vi "RIS.vi"(2 "Run uninterrupted?":bool, 3 "Device Category IN:":string(combo)="Short Strip" caption="Device Category:", 4 "Structure:":string, 5 "DB Serial No.:":string, 6 "Sensor Serial No.:":string) -> (0 "Done!":bool)   [LabVIEW 2019]
doc: "Performs Ris measurements according to ATLAS ITk Quality Control Specifications."
uses:
  <vilib>/Analysis/6fits.llb/Curve Fitting Criteria.ctl
  general_VIs/globals/QC_MeasurementSetup.vi
  general_VIs/globals/QC_RunInformation.vi
  InstrControl/InstrumentSetup.vi
  InstrControl/Switching/Switching.lvclass
  InstrControl/SupplyControl/SupplyControl.lvclass
  InstrControl/MultimeterControl/MultimeterControl.lvclass
  InstrControl/ArduinoControl/ArduinoControl.lvclass
  <vilib>/Analysis/NI_AALBase.lvlib
  InstrControl/InstrControl.lvclass
  <vilib>/Analysis/NI_AALPro.lvlib
panel:
  out "Ris":dbl[](array[numeric]) caption="Ris [MOhm]"
  out "Volts":dbl[](array[numeric]) caption="Volts [V]"
  out "Current":dbl[](array[numeric]) caption="Current [nA]"
  in  "No. of readouts":i32=5
  out "Risgraph":cluster{dbl[], dbl[]}(graph)
  out "Vigraph":cluster{i32[], dbl[]}[](graph)
  out "Imgraph":cluster{i32[], dbl[]}[](graph)
  in  "Initial volts [V]":dbl format="%.1f"
  in  "Final volts [V]":dbl=-700.0 format="%.1f"
  in  "step [V]":dbl=10.0 format="%.1f"
  in  "step interval [s]":u32=10
  out "Temp.":dbl[](array[numeric]) caption="Temp. [°C]" format="%#.2f"
  out "RH":dbl[](array[numeric]) caption="RH [%]" format="%#.2f"
  out "positive ramp?":bool
  out "Tab Control":enum32{"Ris Setup", "Ris Scan"}(tab)
  in  "Switching":string(combo)="Pickering Matrix"
  in  "Voltmeter":string(combo)="HP34401A"
  in  "Ris SMU":string(combo)="Keithley 2657A"
  in  "Current Limit [µA]":dbl=20.0 min=0.0001 format="%.3f"
  in  "Set\ncurrent\nlimit?":bool
  in  "Temperature":enum16{"Read Arduino", "Enter manually"}(ring)
  in  "Ris Supply":string(combo)="Keithley 2410"
  in  "User:":string(combo)="Graham"
  in  "Manufacturer:":string(combo)="Hamamatsu"
  in  "Quit":bool
  in  "Continue":bool
  in  "abort":bool
  out "Device Category:":string
  out "DB Serial Number:":string
  out "Current Volts:":dbl format="%.2f"
  in  "quit (no save)":bool
  in  "Quit & Save":bool
  out "Bias On/Off:":bool
  out "STATUS 1":string
  out "Initiated:":string
  out "Sensor No.:":string
  out "No of steps":u32
  out "Current reading No.":u32
  out "Last reading at:":string
  out "Ris SMU Current [nA]":dbl[][][](array[numeric])
  out "Ris induced Voltage [V]":dbl[][][](array[numeric])
  # "University of\nCambridge"
  # "Strip Sensor QC: inter-strip Resistance"
  # "Ris Scan parameters:"
  # "Last 5 readings:"
  # "n-4"
  # "n-3"
  # "n-2"
  # "n-1"
  # "n"
  # "DUT & Test Description"
  # "Hardware"
  # "DUT & Test Description:"
  # "Current status:"
  # "Rdg No:"
  # "out of"
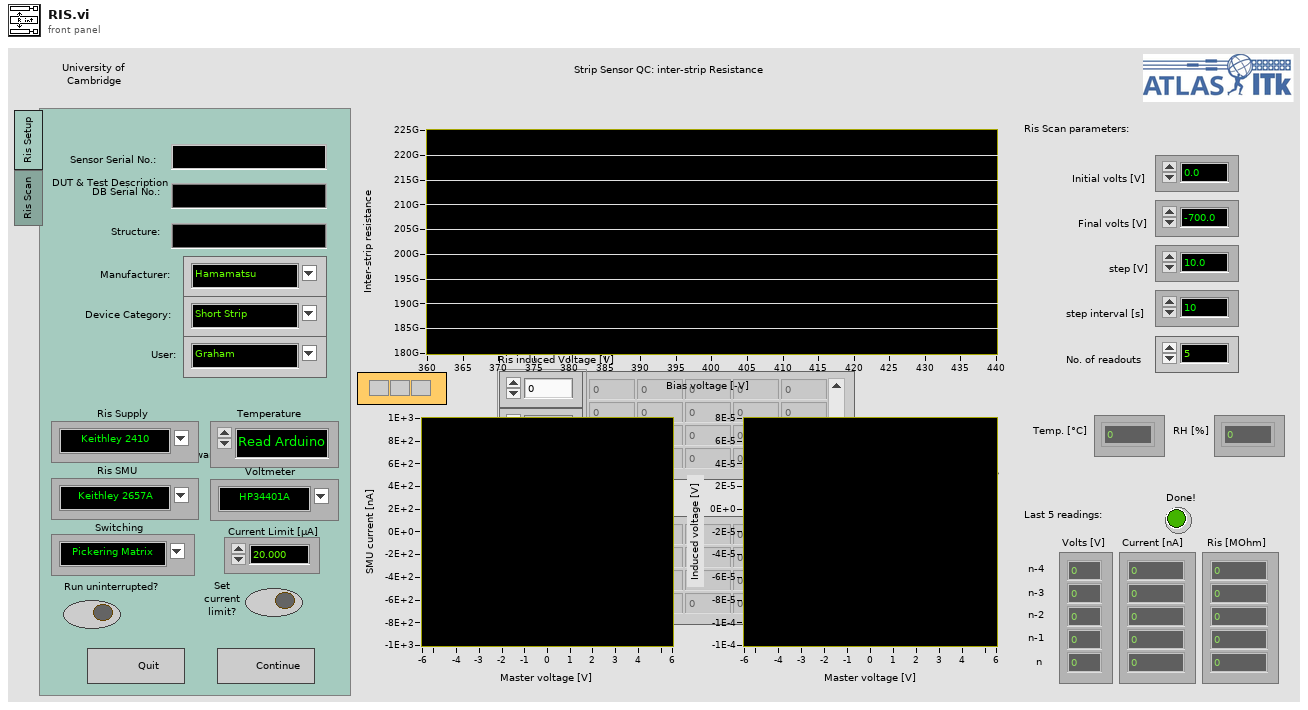
[diagram p1: front panel]
types:
  T1 = enum16{"Supply", "LCR", "Multimeter", "Switching"}
  T2 = enum16{"Reset", "Read Array", "Read Element", "Write Element", "Write Array", "Add Element", "Add Array"}
  T3 = enum16{"Reset", "Ground", "Striptest Bias", "Striptest SMU", "Striptest LCR", "IV", "CV", "Interstrip Cap", "Interstrip Res"}
  T4 = enum16{"Reset", "Ground", "Striptest Bias", "Striptest SMU", "Striptest LCR", "IV", "CV", "Interstrip Cap", "Interstrip Res", "PTP", "Implant Resistance", "Metal Resistance", "Coupling Capacitance"}
  T5 = enum32{"IV", "CV", "Stability", "Striptest", "Cis", "Ris", "PTP"}
  T6 = cluster{"Sensor Serial No.:":string, "Wafer Serial No.:":string, "Batch:":string, "Manufacturer:":string, "Device Category:":string, "Database Serial No.:":string, "Date Initiated:":string, "Time Initiated:":string, "Test":string, "Instruments used:":string, "Probeplan used:":string, "End of Run comment:":string, "User:":string}
  T7 = cluster{"Institute":string, "Manufacturers":string[], "Devices":string[], "Serialnumbers Lookup DB":string, "Data directory":string, "Backup & screenshot directory":string, "List of known users":string[], "Measurement switch not used":bool, "Measurement Switch":string, "DUT Switch":string}
  T8 = cluster{"Bias Supply":refnum<class "SupplyControl.lvclass">, "SMU":refnum<class "SupplyControl.lvclass">, "Multimeter":refnum<class "MultimeterControl.lvclass">, "Initial Voltage [V]":dbl, "Final Voltage [V]":dbl, "Step Size [V]":dbl, "Step Interval [s]":i32, "Number Of Steps":u32, "Ramp down steps [V]":dbl, "Ramp down Interval [s]":i32, "Set Current Limit?":bool, "Current Limit [µA]":dbl, "Temperature Readout":enum16{"Read Arduino", "Enter manually"}, "Arduino":refnum<class "ArduinoControl.lvclass">, "Supply Name":string, "SMU Name":string, "Voltmeter Name":string, "R_is Limit [MOhm]":dbl, "Switching":refnum<class "Switching.lvclass">, "Matrix used?":bool, "Matrix X Channels":cluster{"Bias Supply / SMU LO":i32, "Bias Supply / SMU HI":i32, "CV Box LO":i32, "CV Box HI":i32, "CV Box LO IN":i32, "CV Box HI IN":i32, "Volt meter LO":i32, "Volt meter HI":i32, "Mux1 C1":i32, "Mux1 C2":i32, "Mux2 C1":i32, "Mux2 C2":i32}, "Structure Name":string}
  T9 = cluster{"Current Limit":sgl, "KE2410":refnum<class "KE2410.lvclass">}
  T10 = cluster{"VISA address":refnum<visa-resource-name>, "T sensor":enum16{"SHT", "DS"}, "Arduino":refnum<class "ArduinoControl.lvclass">}
  T11 = typedef "NI_AALPro.lvlib/Curve Fitting Criteria.ctl" = u16
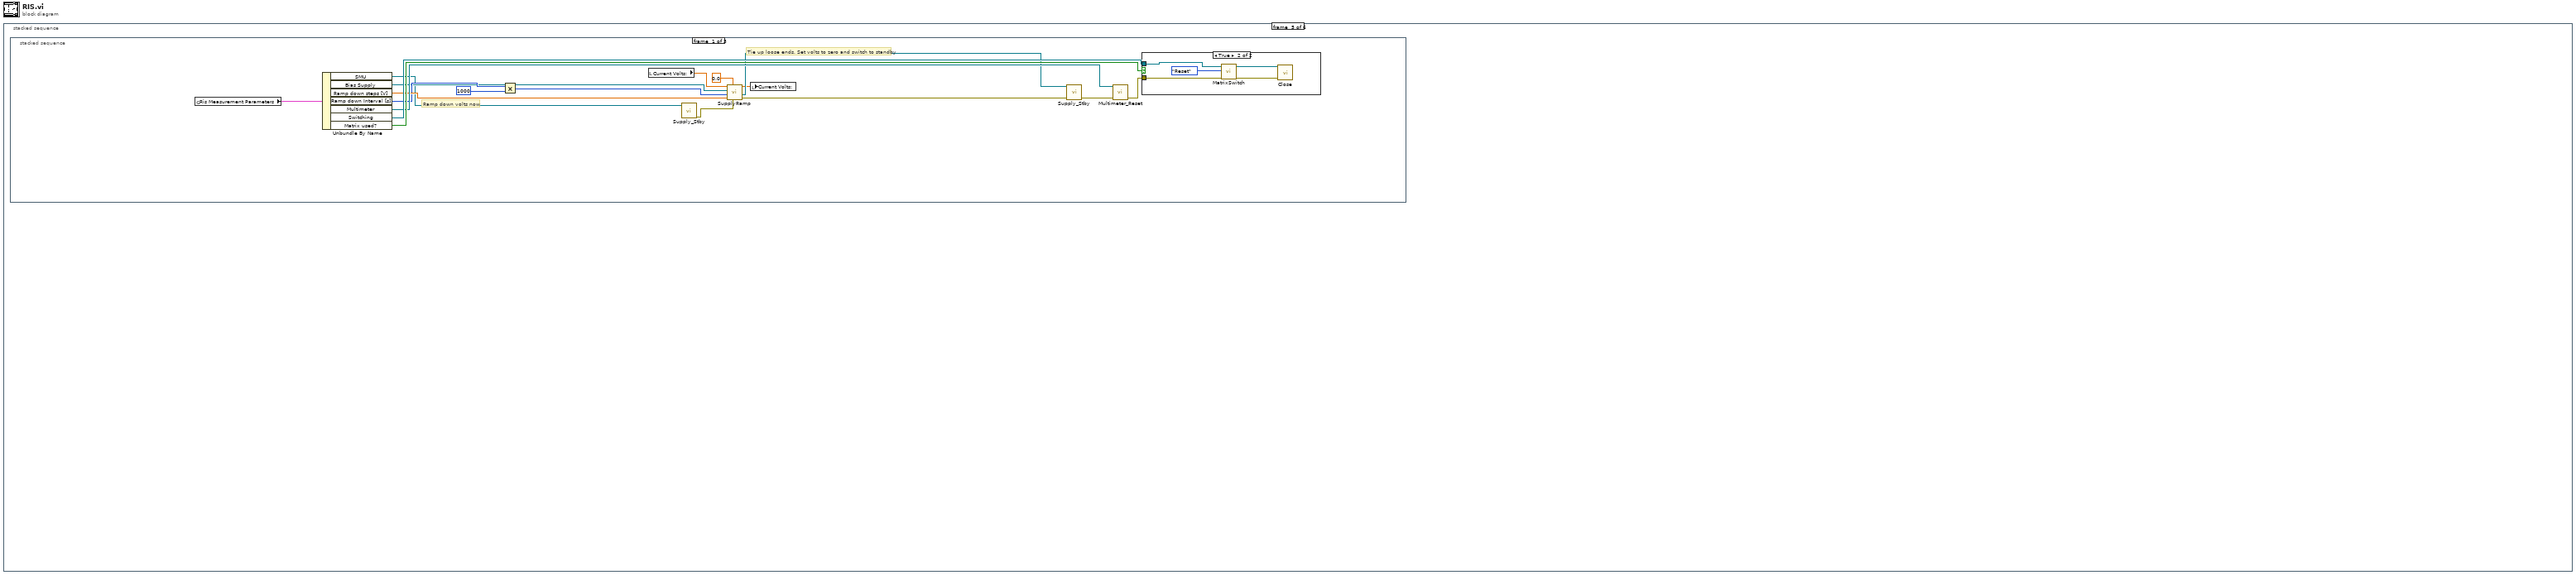
[diagram p0: block diagram]
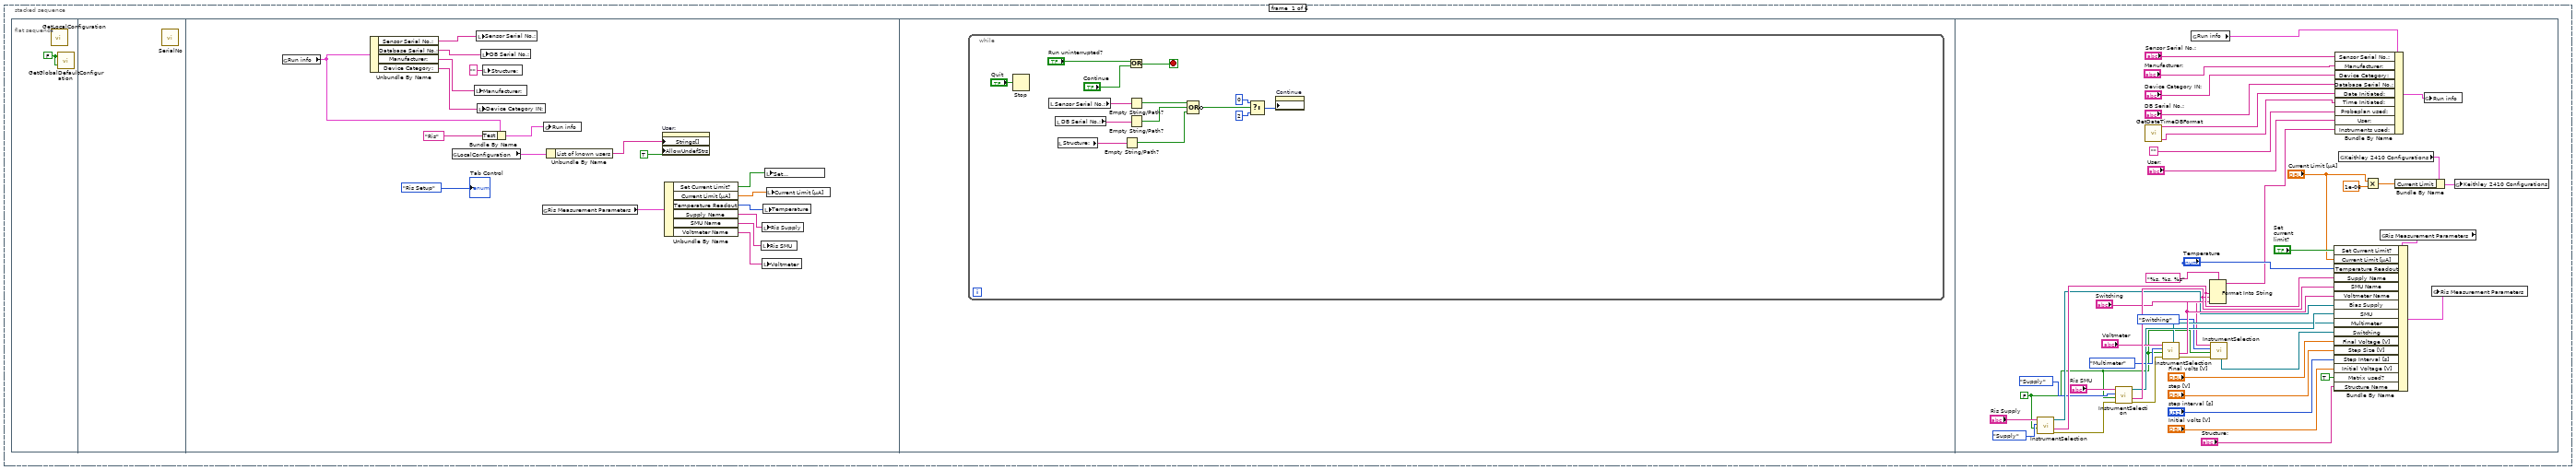
[diagram p2: hidden frame]
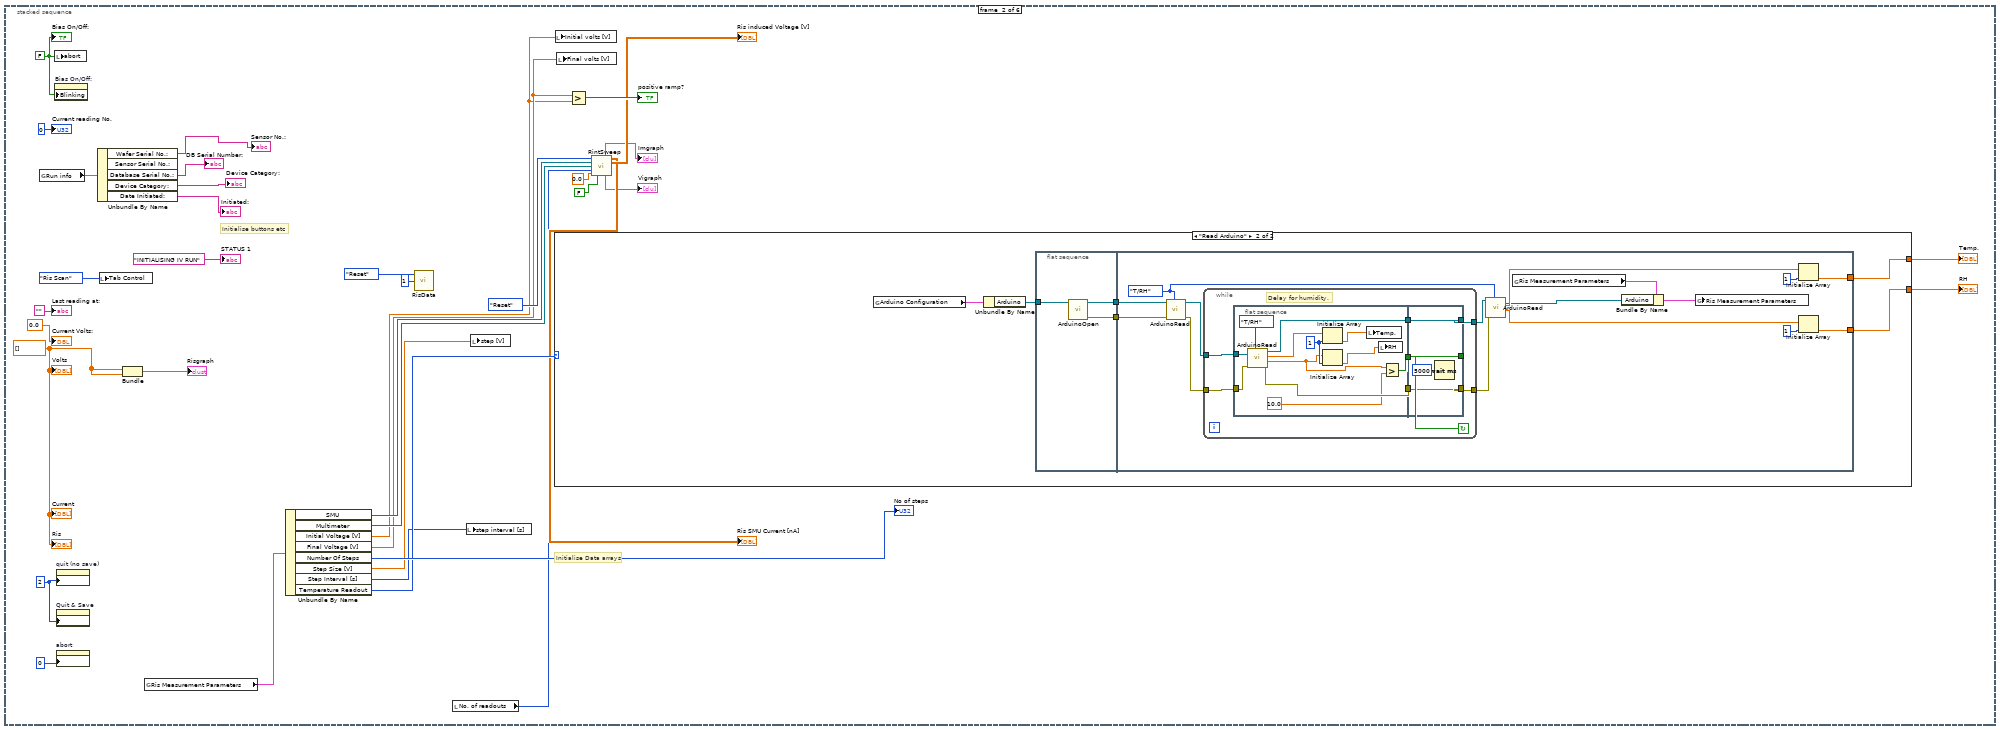
[diagram p3: hidden frame]
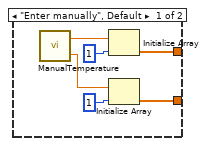
[diagram p4: hidden frame]
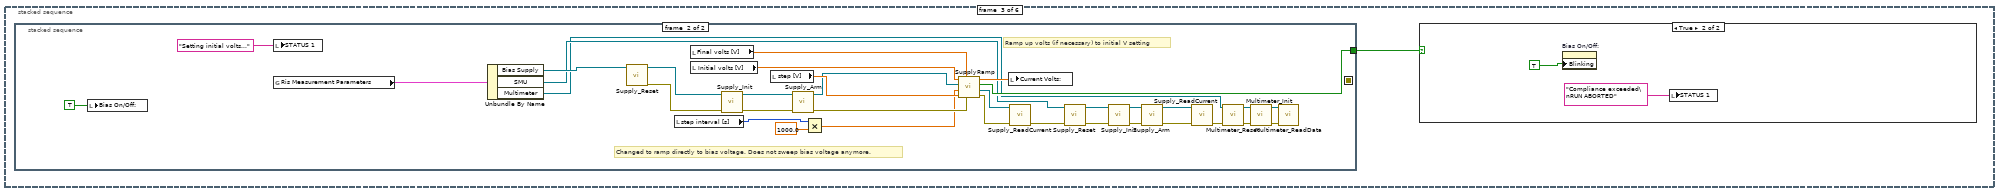
[diagram p5: hidden frame]
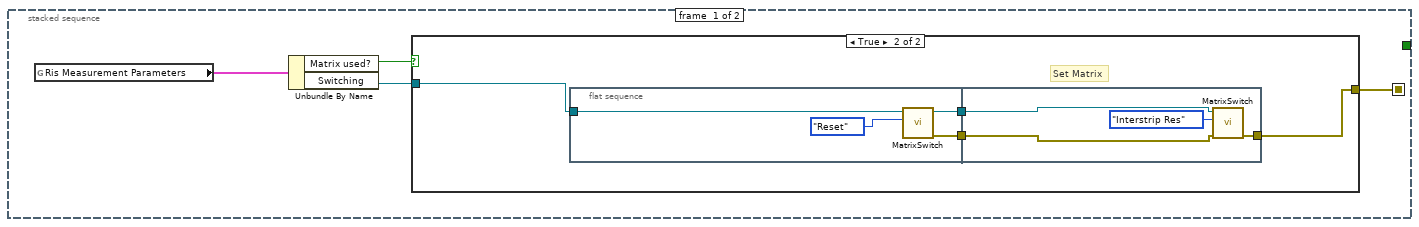
[diagram p6: hidden frame]
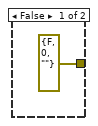
[diagram p7: hidden frame]
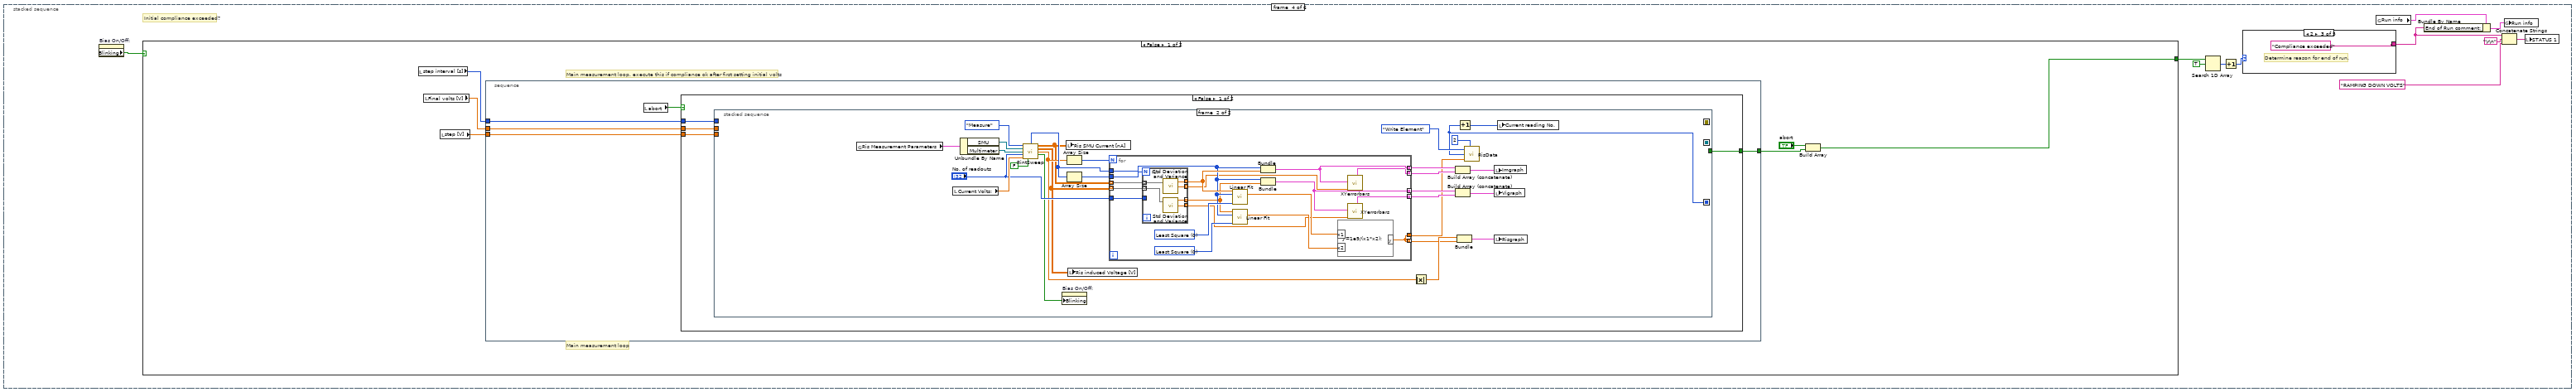
[diagram p9: hidden frame]
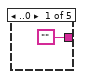
[diagram p10: hidden frame]
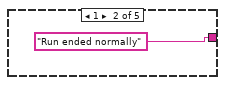
[diagram p11: hidden frame]
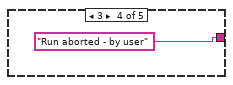
[diagram p12: hidden frame]
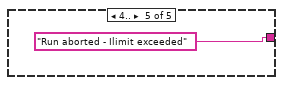
[diagram p13: hidden frame]
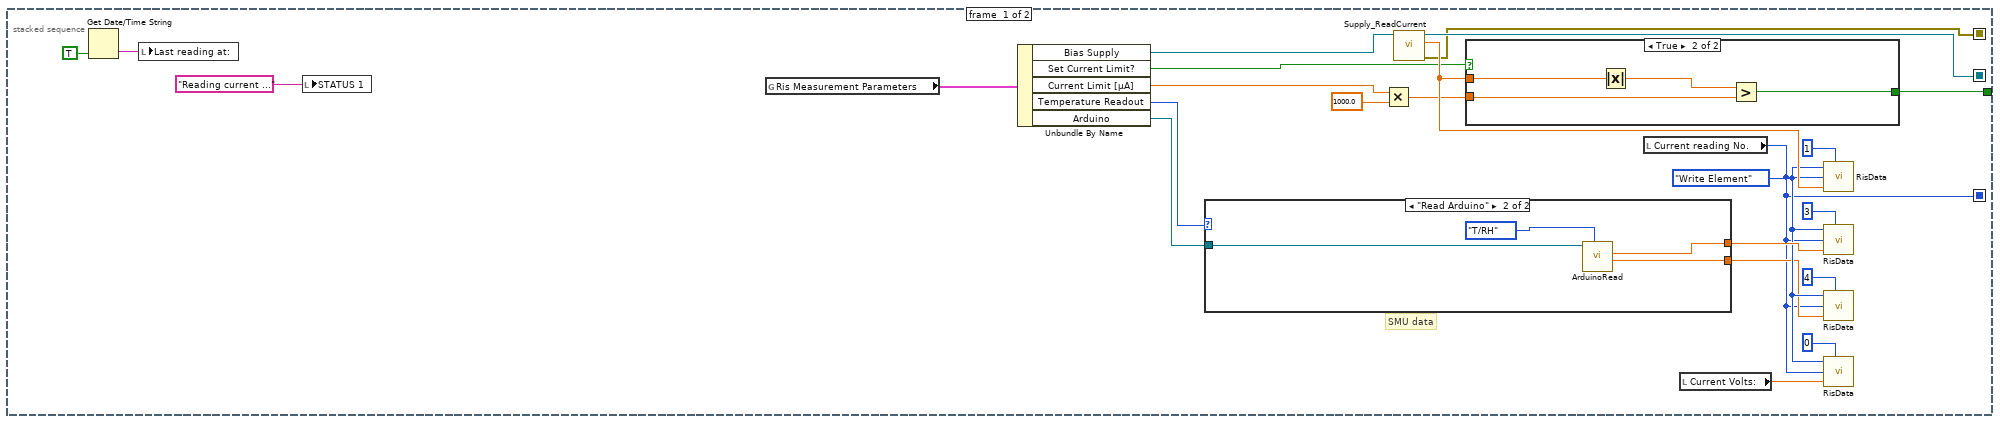
[diagram p14: hidden frame]
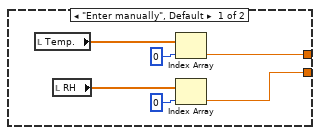
[diagram p15: hidden frame]
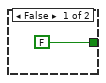
[diagram p16: hidden frame]
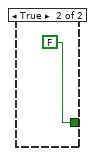
[diagram p17: hidden frame]
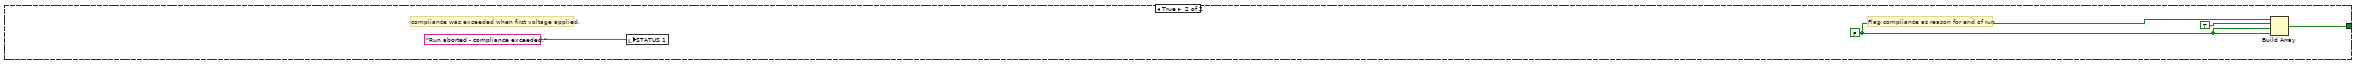
[diagram p18: hidden frame]
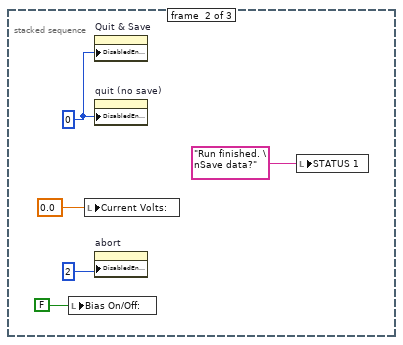
[diagram p20: hidden frame]
diagram:
  n1 = stacked-sequence {
    frame #0 {
      n2 = flat-sequence {
        frame #0 {
          w1 = FALSE
          n3 = call "GetLocalConfiguration.vi"() -> ()  [unwired: 3 in, 1 out]
          n4 = call "GetGlobalDefaultConfiguration.vi"("DO NOT override instruments"=w1, "Read defaults?"=w1) -> ()  [unwired: 1 in, 1 out]
        }
        frame #1 {
          n5 = call "SerialNo.vi"() -> ()  [unwired: 5 in, 1 out]
        }
        frame #2 {
          n6 = global read "QC_RunInformation.vi" "Run info"() -> (w7:T6)
          n7 = Unbundle By Name(w7) -> ("Sensor Serial No.:"=w4:string, "Database Serial No.:"=w5:string, "Manufacturer:"=w3:string, "Device Category:"=w6:string)
          n8 = global read "QC_RunInformation.vi" "LocalConfiguration"() -> (w15:T7)
          n9 = local write "Manufacturer:"(w3) -> ()
          n10 = local write "Sensor Serial No.:"(w4) -> ()
          n11 = local write "Device Category IN:"(w6) -> ()
          n12 = local write "DB Serial No.:"(w5) -> ()
          n13 = local write "Structure:"("" ("Structure:")) -> ()
          n14 = Bundle By Name(cluster=w7, "Test"="Ris") -> (w12:T6)
          n15 = global read "QC_MeasurementSetup.vi" "Ris Measurement Parameters"() -> (w18:T8)
          n16 = global write "QC_RunInformation.vi" "Run info"(w12) -> ()
          n17 = Unbundle By Name(w15) -> ("List of known users"=w14:string[])
          n18 = property on="User:" class="CmbBox"("Strings[]"=w14, "AllowUndefStrs"=TRUE) -> ()  [unwired: 2 in, 2 out]
          n19 = Unbundle By Name(w18) -> ("Set Current Limit?"=w17:bool, "Current Limit [µA]"=w16:dbl, "Temperature Readout"=w20:enum16{"Read Arduino", "Enter manually"}, "Supply Name"=w19:string, "SMU Name"=w9:string, "Voltmeter Name"=w8:string)
          n20 = local write "Ris SMU"(w9) -> ()
          n21 = local write "Ris Supply"(w19) -> ()
          n22 = local write "Voltmeter"(w8) -> ()
          n23 = local write "Temperature"(w20) -> ()
          n24 = local write "Set\ncurrent\nlimit?"(w17) -> ()
          n25 = local write "Current Limit [µA]"(w16) -> ()
          "Tab Control" <- enum32{"Ris Setup", "Ris Scan"}."Ris Setup" ("Tab Control")
        }
        frame #3 {
          n26 = while {
            stop <- w23 stop-if-true
            n27 = Stop(stop? (T)="Quit") -> ()
            n28 = local read "Sensor Serial No.:"() -> (w33:string)
            n29 = local read "DB Serial No.:"() -> (w32:string)
            n30 = local read "Structure:"() -> (w22:string)
            n31 = Empty String/Path?(string/path=w22) -> (empty?=w21:bool)
            n32 = Or(x="Run uninterrupted?", y="Continue") -> (x .or. y?=w23:bool)
            n33 = Empty String/Path?(string/path=w33) -> (empty?=w30:bool)
            n34 = Empty String/Path?(string/path=w32) -> (empty?=w31:bool)
            n35 = Compound Arithmetic op=OR(w30, w31, w21) -> (invert w29:bool)
            n36 = Select(t=0, s=w29, f=2) -> (s? t:f=w26:i32)
            n37 = property on="Continue" class="Bool"("DisabledEnum"=w26) -> ()  [unwired: 2 in, 2 out]
          }
        }
        frame #4 {
          w52 = FALSE
          n38 = call "InstrumentSelection.vi"("Verify GPIB address"=w52, "Instrument type"=T1."Supply", "Instrument name IN"="Ris Supply") -> ("error out"=w59:errorcluster, "Instrument name OUT"=w67:string, "Supply"=w62:refnum<class "SupplyControl.lvclass">)  [unwired: 3 in, 3 out]
          n39 = call "InstrumentSelection.vi"("error in (no error)"=w59, "Verify GPIB address"=w52, "Instrument type"=T1."Supply", "Instrument name IN"="Ris SMU") -> ("error out"=w58:errorcluster, "Instrument name OUT"=w65:string, "Supply"=w61:refnum<class "SupplyControl.lvclass">)  [unwired: 2 in, 3 out]
          n40 = call "GetDateTimeDBFormat.vi"() -> ("Time in 24h format, e.g. 13:40:54"=w36:string, "Abbreviated Date, e.g. 13 Nov 2020"=w38:string)  [unwired: 10 in]
          n41 = call "InstrumentSelection.vi"("error in (no error)"=w58, "Verify GPIB address"=w52, "Instrument type"=T1."Multimeter", "Instrument name IN"="Voltmeter") -> ("error out"=w57:errorcluster, "Instrument name OUT"=w63:string, "Multimeter"=w60:refnum<class "MultimeterControl.lvclass">)  [unwired: 2 in, 3 out]
          n42 = global read "QC_RunInformation.vi" "Run info"() -> (w78:T6)
          n43 = Format Into String(format string="%s, %s, %s", w67, w65, w63) -> (resulting string=w35:string)  [unwired: 2 in, 1 out]
          n44 = call "InstrumentSelection.vi"("error in (no error)"=w57, "Verify GPIB address"=w52, "Instrument type"=T1."Switching", "Instrument name IN"="Switching") -> ("Switching"=w51:refnum<class "Switching.lvclass">)  [unwired: 2 in, 5 out]
          n45 = Bundle By Name(cluster=w78, "Sensor Serial No.:"="Sensor Serial No.:", "Manufacturer:"="Manufacturer:", "Device Category:"="Device Category IN:", "Database Serial No.:"="DB Serial No.:", "Date Initiated:"=w38, "Time Initiated:"=w36, "Probeplan used:"="", "User:"="User:", "Instruments used:"=w35) -> (w77:T6)
          n46 = global read "InstrumentSetup.vi" "Keithley 2410 Configurations"() -> (w43:T9)
          n47 = Multiply(x="Current Limit [µA]", y=1e-06) -> (x*y=w40:dbl)
          n48 = global read "QC_MeasurementSetup.vi" "Ris Measurement Parameters"() -> (w79:T8)
          n49 = Bundle By Name(cluster=w79, "Set Current Limit?"="Set\ncurrent\nlimit?", "Current Limit [µA]"="Current Limit [µA]", "Temperature Readout"="Temperature", "Supply Name"=w67, "SMU Name"=w65, "Voltmeter Name"=w63, "Bias Supply"=w62, "SMU"=w61, "Multimeter"=w60, "Switching"=w51, "Final Voltage [V]"="Final volts [V]", "Step Size [V]"="step [V]", "Step Interval [s]"="step interval [s]", "Initial Voltage [V]"="Initial volts [V]", "Matrix used?"=TRUE, "Structure Name"="Structure:") -> (w80:T8)
          n50 = Bundle By Name(cluster=w43, "Current Limit"=w40) -> (w44:T9)
          n51 = global write "QC_RunInformation.vi" "Run info"(w77) -> ()
          n52 = global write "QC_MeasurementSetup.vi" "Ris Measurement Parameters"(w80) -> ()
          n53 = global write "InstrumentSetup.vi" "Keithley 2410 Configurations"(w44) -> ()
        }
      }
    }
    frame #1 {
      w92 = dbl[] []
      w108 = 2
      w107 = FALSE ("Visible")
      # "Initialise buttons etc"
      # "Initialise Data arrays"
      n54 = global read "QC_RunInformation.vi" "Run info"() -> (w116:T6)
      n55 = local write "abort"(w107) -> ()
      n56 = property on="Bias On/Off:" class="Bool (strict)"("Blinking"=w107) -> ()  [unwired: 2 in, 2 out]
      n57 = property on="quit (no save)" class="Bool"("DisabledEnum"=w108) -> ()  [unwired: 2 in, 2 out]
      n58 = property on="Quit & Save" class="Bool"("DisabledEnum"=w108) -> ()  [unwired: 2 in, 2 out]
      n59 = property on="abort" class="Bool (strict)"("DisabledEnum"=0) -> ()  [unwired: 2 in, 2 out]
      n60 = Unbundle By Name(w116) -> ("Wafer Serial No.:"=→"Sensor No.:":string, "Database Serial No.:"=→"DB Serial Number:":string, "Device Category:"=→"Device Category:":string, "Date Initiated:"=→"Initiated:":string)  [unwired: 1 out]
      n61 = local write "Tab Control"(enum32{"Ris Setup", "Ris Scan"}."Ris Scan" ("Tab Control")) -> ()
      n62 = Bundle(w92, w92) -> (→"Risgraph":cluster{dbl[], dbl[]})  [unwired: 1 in]
      n63 = global read "QC_MeasurementSetup.vi" "Ris Measurement Parameters"() -> (w103:T8)
      n64 = Unbundle By Name(w103) -> ("SMU"=w88:refnum<class "SupplyControl.lvclass">, "Multimeter"=w87:refnum<class "MultimeterControl.lvclass">, "Initial Voltage [V]"=w83:dbl, "Final Voltage [V]"=w84:dbl, "Number Of Steps"=→"No of steps":u32, "Step Size [V]"=w85:dbl, "Step Interval [s]"=w86:i32, "Temperature Readout"=w109:enum16{"Read Arduino", "Enter manually"})
      n65 = call "RisData.vi"("Action"=T2."Reset", "Array Size / Index"=u32 1) -> ()  [unwired: 3 in, 2 out]
      n66 = local read "No. of readouts"() -> (w90:i32)
      n67 = local write "step interval [s]"(w86) -> ()
      n68 = local write "step [V]"(w85) -> ()
      n69 = case shown="\"Read Arduino\"" w109 {
        tunnel: [w122 w129] -> w111
        tunnel: [w119 w128] -> w104
        frame "Enter manually", Default {
          n70 = call "ManualTemperature.vi"() -> ("Humidity [%] out"=w118:dbl, "Temperature [°C] out"=w123:dbl)
          n71 = Initialize Array(w123, 1) -> (w122:dbl[])
          n72 = Initialize Array(w118, 1) -> (w119:dbl[])
        }
        frame "Read Arduino" {
          n73 = global read "InstrumentSetup.vi" "Arduino Configuration"() -> (w125:T10)
          n74 = Unbundle By Name(w125) -> ("Arduino"=w124:refnum<class "ArduinoControl.lvclass">)
          n75 = flat-sequence {
            tunnel: [w130] -> w127
            tunnel: [w132] -> w126
            tunnel: w124 -> [w131]
            tunnel: [w148] -> w129
            tunnel: [w145] -> w128
            tunnel: w127 -> [w139]
            tunnel: w126 -> [w138]
            frame #0 {
              n76 = call "ArduinoOpen.vi"("ArduinoControl in"=w131) -> ("error out"=w132:errorcluster, "ArduinoControl out"=w130:refnum<class "ArduinoControl.lvclass">)  [unwired: 9 in]
            }
            frame #1 {
              w137 = enum16{"T/RH", "Interlock", "Edgesense"}."T/RH" ("Arduino function")
              n77 = call "ArduinoRead.vi"("Arduino function"=w137, "error in (no error)"=w138, "ArduinoControl in"=w139) -> ("error out"=w135:errorcluster, "ArduinoControl out"=w136:refnum<class "ArduinoControl.lvclass">)  [unwired: 3 in, 4 out]
              n78 = while {
                tunnel: w136 -> [w156]
                tunnel: w135 -> [w155]
                tunnel: [w153] -> w134
                tunnel: [w152] -> w133
                stop <- w154 continue-if-true
                # "Delay for humidity."
                n79 = flat-sequence {
                  tunnel: w156 -> [w168]
                  tunnel: w155 -> [w166]
                  tunnel: [w165] -> w151
                  tunnel: [w164] -> w150
                  tunnel: [w163] -> w149
                  tunnel: [w170] -> w152
                  tunnel: [w171] -> w153
                  tunnel: [w172] -> w154
                  tunnel: w151 -> [w172]
                  tunnel: w150 -> [w171]
                  tunnel: w149 -> [w170]
                  frame #0 {
                    w161 = 1
                    n80 = call "ArduinoRead.vi"("Arduino function"=enum16{"T/RH", "Interlock", "Edgesense"}."T/RH", "error in (no error)"=w166, "ArduinoControl in"=w168) -> ("error out"=w163:errorcluster, "rel. Humidity [%]"=w158:dbl, "Temperature [°C]"=w159:dbl, "ArduinoControl out"=w164:refnum<class "ArduinoControl.lvclass">)  [unwired: 3 in, 2 out]
                    n81 = Initialize Array(w159, w161) -> (w160:dbl[])
                    n82 = Initialize Array(w158, w161) -> (w157:dbl[])
                    n83 = local write "Temp."(w160) -> ()
                    n84 = local write "RH"(w157) -> ()
                    n85 = Greater?(x=w158, y=10.0 ("Start Humidity")) -> (0:w165:bool)
                  }
                  frame #1 {
                    n86 = Wait (ms)(milliseconds to wait=u32 5000) -> ()  [unwired: 1 out]
                  }
                }
              }
              n87 = call "ArduinoRead.vi"("Arduino function"=w137, "error in (no error)"=w133, "ArduinoControl in"=w134) -> ("rel. Humidity [%]"=w143:dbl, "Temperature [°C]"=w144:dbl, "ArduinoControl out"=w142:refnum<class "ArduinoControl.lvclass">)  [unwired: 3 in, 3 out]
              n88 = global read "QC_MeasurementSetup.vi" "Ris Measurement Parameters"() -> (w141:T8)
              n89 = Bundle By Name(cluster=w141, "Arduino"=w142) -> (w140:T8)
              n90 = global write "QC_MeasurementSetup.vi" "Ris Measurement Parameters"(w140) -> ()
              n91 = Initialize Array(w144, 1) -> (w148:dbl[])
              n92 = Initialize Array(w143, 1) -> (w145:dbl[])
            }
          }
        }
      }
      "Temp." <- w111
      "RH" <- w104
      n93 = local write "Initial volts [V]"(w83) -> ()
      n94 = local write "Final volts [V]"(w84) -> ()
      n95 = Greater?(x=w84, y=w83) -> (0:→"positive ramp?":bool)
      n96 = call "RintSweep.vi"("Action"=enum16{"Reset", "Measure"}."Reset", "MasterVoltage Supply in"=w88, "VoltmeterControl in"=w87, "No. of readouts"=w90, "Bias [V]"=0.0, "Simulated data?"=FALSE) -> ("Igraph"=→"Imgraph":cluster{i32[], dbl[]}[], "Applied Current [nA]"=→"Ris SMU Current [nA]":dbl[][][], "Induced Voltage [V]"=→"Ris induced Voltage [V]":dbl[][][], "ViGraph"=→"Vigraph":cluster{i32[], dbl[]}[])  [unwired: 2 in, 4 out]
      "STATUS 1" <- "INITIALISING IV RUN"
      "Bias On/Off:" <- w107
      "Last reading at:" <- ""
      "Current reading No." <- u32 0 ("Current reading No.")
      "Current Volts:" <- 0.0 ("Current Volts:")
      "Current" <- w92
      "Volts" <- w92
      "Ris" <- w92
    }
    frame #2 {
      n97 = stacked-sequence {
        seq-local: [w175 _] -> [_ _]
        tunnel: [_ w210] -> w173
        frame #0 {
          n98 = global read "QC_MeasurementSetup.vi" "Ris Measurement Parameters"() -> (w174:T8)
          n99 = Unbundle By Name(w174) -> ("Matrix used?"=w177:bool, "Switching"=w176:refnum<class "Switching.lvclass">)
          n100 = case shown="True" w177 {
            tunnel: w176 -> [_ w179]
            tunnel: [errorcluster {"status"=FALSE, "code"=0, "source"=""} ("error constant") w180] -> w175
            frame False {
            }
            frame True {
              # "Set Matrix"
              n101 = flat-sequence {
                tunnel: [w186] -> w182
                tunnel: [w185] -> w181
                tunnel: w179 -> [w184]
                tunnel: w182 -> [w190]
                tunnel: w181 -> [w189]
                tunnel: [w188] -> w180
                frame #0 {
                  n102 = call-dynamic "MatrixSwitch.vi"("Action"=T3."Reset", "Switching in"=w184) -> ("error out"=w186:errorcluster, "Switching out"=w185:refnum<class "Switching.lvclass">)  [unwired: 7 in, 1 out]
                }
                frame #1 {
                  n103 = call-dynamic "MatrixSwitch.vi"("error in (no error)"=w190, "Action"=T4."Interstrip Res", "Switching in"=w189) -> ("error out"=w188:errorcluster)  [unwired: 6 in, 2 out]
                }
              }
            }
          }
        }
        frame #1 {
          # "Changed to ramp directly to bias voltage. Does not sweep bias voltage anymore."
          # "Ramp up volts (if necessary) to initial V setting"
          n104 = local write "Bias On/Off:"(TRUE ("Compliance?")) -> ()
          n105 = local write "STATUS 1"("Setting initial volts..." ("STATUS 1")) -> ()
          n106 = global read "QC_MeasurementSetup.vi" "Ris Measurement Parameters"() -> (w220:T8)
          n107 = Unbundle By Name(w220) -> ("Bias Supply"=w217:refnum<class "SupplyControl.lvclass">, "SMU"=w202:refnum<class "SupplyControl.lvclass">, "Multimeter"=w197:refnum<class "MultimeterControl.lvclass">)
          n108 = call-dynamic "Supply_Reset.vi"("SupplyControl in"=w217) -> ("error out"=w222:errorcluster, "SupplyControl out"=w224:refnum<class "SupplyControl.lvclass">)  [unwired: 9 in]
          n109 = local read "step interval [s]"() -> (w192:u32)
          n110 = local read "Final volts [V]"() -> (w194:dbl)
          n111 = local read "Initial volts [V]"() -> (w195:dbl)
          n112 = call-dynamic "Supply_Init.vi"("error in (no error)"=w222, "SupplyControl in"=w224) -> ("error out"=w221:errorcluster, "SupplyControl out"=w223:refnum<class "SupplyControl.lvclass">)  [unwired: 8 in]
          n113 = local read "step [V]"() -> (w213:dbl)
          n114 = call-dynamic "Supply_Arm.vi"("error in (no error)"=w221, "SupplyControl in"=w223) -> ("error out"=w212:errorcluster, "SupplyControl out"=w211:refnum<class "SupplyControl.lvclass">)  [unwired: 8 in]
          n115 = Multiply(x=w192, y=1000.0) -> (x*y=w191:dbl)
          n116 = call "SupplyRamp.vi"("error in"=w212, "Requested Voltage"=w194, "Step Size"=w213, "Step Delay"=w191, "Supply IN"=w211, "Starting Voltage"=w195) -> ("error out"=w215:errorcluster, "Supply OUT"=w216:refnum<class "SupplyControl.lvclass">, "Compliance exceeded"=w210:bool, "Current Voltage"=w214:dbl)  [unwired: 2 in]
          n117 = local write "Current Volts:"(w214) -> ()
          n118 = call-dynamic "Supply_ReadCurrent.vi"("error in (no error)"=w215, "SupplyControl in"=w216) -> ("error out"=w203:errorcluster)  [unwired: 7 in, 2 out]
          n119 = call-dynamic "Supply_Reset.vi"("error in (no error)"=w203, "SupplyControl in"=w202) -> ("error out"=w207:errorcluster, "SupplyControl out"=w209:refnum<class "SupplyControl.lvclass">)  [unwired: 8 in]
          n120 = call-dynamic "Supply_Init.vi"("error in (no error)"=w207, "SupplyControl in"=w209) -> ("error out"=w206:errorcluster, "SupplyControl out"=w208:refnum<class "SupplyControl.lvclass">)  [unwired: 8 in]
          n121 = call-dynamic "Supply_Arm.vi"("error in (no error)"=w206, "SupplyControl in"=w208) -> ("error out"=w205:errorcluster, "SupplyControl out"=w204:refnum<class "SupplyControl.lvclass">)  [unwired: 8 in]
          n122 = call-dynamic "Supply_ReadCurrent.vi"("error in (no error)"=w205, "SupplyControl in"=w204) -> ("error out"=w196:errorcluster)  [unwired: 7 in, 2 out]
          n123 = call-dynamic "Multimeter_Reset.vi"("error in (no error)"=w196, "MultimeterControl in"=w197) -> ("error out"=w198:errorcluster, "MultimeterControl out"=w199:refnum<class "MultimeterControl.lvclass">)  [unwired: 8 in]
          n124 = call-dynamic "Multimeter_Init.vi"("error in (no error)"=w198, "MultimeterControl in"=w199) -> ("error out"=w201:errorcluster, "MultimeterControl out"=w200:refnum<class "MultimeterControl.lvclass">)  [unwired: 8 in]
          n125 = call-dynamic "Multimeter_ReadData.vi"("error in (no error)"=w201, "MultimeterControl in"=w200) -> ()  [unwired: 7 in, 3 out]
        }
      }
      n126 = case shown="True" w173 {
        frame False {
        }
        frame True {
          n127 = property on="Bias On/Off:" class="Bool (strict)"("Blinking"=TRUE) -> ()  [unwired: 2 in, 2 out]
          n128 = local write "STATUS 1"("Compliance exceeded\nRUN ABORTED") -> ()
        }
      }
    }
    frame #3 {
      # "Initial compliance exceeded?"
      n129 = property on="Bias On/Off:" class="Bool (strict)"() -> ("Blinking"=w237:bool)  [unwired: 2 in, 2 out]
      n130 = case shown="False" w237 {
        tunnel: [w248 w351] -> w236
        frame False {
          # "Main measurement loop"
          # "Main measurement loop. execute this if compliance ok after first setting initial volts"
          n131 = local read "step interval [s]"() -> (w245:u32)
          n132 = local read "Final volts [V]"() -> (w246:dbl)
          n133 = local read "step [V]"() -> (w247:dbl)
          n134 = stacked-sequence {
            tunnel: w247 -> [w253]
            tunnel: w246 -> [w252]
            tunnel: w245 -> [w251]
            tunnel: [w249] -> w244
            frame #0 {
              n135 = local read "abort"() -> (w250:bool)
              n136 = case shown="False" w250 {
                tunnel: w251 -> [w257 _]
                tunnel: w252 -> [w256 _]
                tunnel: w253 -> [w255 _]
                tunnel: [w254 FALSE] -> w249
                frame False {
                  n137 = stacked-sequence {
                    seq-local: [w258 _] -> [_ w298]
                    seq-local: [w268 _] -> [_ _]
                    seq-local: [w267 _] -> [_ _]
                    tunnel: w255 -> [_ _]
                    tunnel: w256 -> [_ _]
                    tunnel: w257 -> [_ _]
                    tunnel: [w275 _] -> w254
                    frame #0 {
                      w270 = T2."Write Element" ("Action")
                      # "SMU data"
                      n138 = Get Date/Time String(want seconds? (F)=TRUE) -> (time string=w272:string)  [unwired: 2 in, 1 out]
                      n139 = local write "Last reading at:"(w272) -> ()
                      n140 = local write "STATUS 1"("Reading current ..." ("status")) -> ()
                      n141 = global read "QC_MeasurementSetup.vi" "Ris Measurement Parameters"() -> (w266:T8)
                      n142 = Unbundle By Name(w266) -> ("Bias Supply"=w260:refnum<class "SupplyControl.lvclass">, "Set Current Limit?"=w265:bool, "Current Limit [µA]"=w262:dbl, "Temperature Readout"=w264:enum16{"Read Arduino", "Enter manually"}, "Arduino"=w259:refnum<class "ArduinoControl.lvclass">)
                      n143 = case shown="\"Read Arduino\"" w264 {
                        tunnel: [w285 w291] -> w273
                        tunnel: [w282 w290] -> w269
                        tunnel: w259 -> [_ w289]
                        frame "Enter manually", Default {
                          n144 = local read "Temp."() -> (w287:dbl[])
                          n145 = local read "RH"() -> (w283:dbl[])
                          n146 = Index Array(array=w287, index=0) -> (element=w285:dbl)
                          n147 = Index Array(array=w283, index=0) -> (element=w282:dbl)
                        }
                        frame "Read Arduino" {
                          n148 = call "ArduinoRead.vi"("Arduino function"=enum16{"T/RH", "Interlock", "Edgesense"}."T/RH", "ArduinoControl in"=w289) -> ("rel. Humidity [%]"=w290:dbl, "Temperature [°C]"=w291:dbl)  [unwired: 4 in, 4 out]
                        }
                      }
                      n149 = Multiply(x=w262, y=1000.0) -> (x*y=w261:dbl)
                      n150 = call-dynamic "Supply_ReadCurrent.vi"("SupplyControl in"=w260) -> ("error out"=w267:errorcluster, "Current in nA"=w276:dbl, "SupplyControl out"=w268:refnum<class "SupplyControl.lvclass">)  [unwired: 8 in]
                      n151 = case shown="True" w265 {
                        tunnel: w276 -> [_ w296]
                        tunnel: w261 -> [_ w294]
                        tunnel: [FALSE w293] -> w275
                        frame False {
                        }
                        frame True {
                          n152 = Absolute Value(x=w296) -> (abs(x)=w295:dbl)
                          n153 = Greater?(x=w295, y=w294) -> (0:w293:bool)
                        }
                      }
                      n154 = local read "Current reading No."() -> (w258:u32)
                      n155 = local read "Current Volts:"() -> (w277:dbl)
                      n156 = call "RisData.vi"("Action"=w270, "Array No."=u32 1, "Array Size / Index"=w258, "Data IN"=w276) -> ()  [unwired: 1 in, 2 out]
                      n157 = call "RisData.vi"("Action"=w270, "Array No."=u32 3, "Array Size / Index"=w258, "Data IN"=w273) -> ()  [unwired: 1 in, 2 out]
                      n158 = call "RisData.vi"("Action"=w270, "Array No."=u32 4, "Array Size / Index"=w258, "Data IN"=w269) -> ()  [unwired: 1 in, 2 out]
                      n159 = call "RisData.vi"("Action"=w270, "Array No."=0, "Array Size / Index"=w258, "Data IN"=w277) -> ()  [unwired: 1 in, 2 out]
                    }
                    frame #1 {
                      n160 = global read "QC_MeasurementSetup.vi" "Ris Measurement Parameters"() -> (w317:T8)
                      n161 = local read "Current Volts:"() -> (w320:dbl)
                      n162 = Unbundle By Name(w317) -> ("SMU"=w316:refnum<class "SupplyControl.lvclass">, "Multimeter"=w315:refnum<class "MultimeterControl.lvclass">)
                      n163 = call "RintSweep.vi"("Action"=enum16{"Reset", "Measure"}."Measure", "MasterVoltage Supply in"=w316, "VoltmeterControl in"=w315, "No. of readouts"="No. of readouts", "Bias [V]"=w320, "Simulated data?"=FALSE) -> ("Sweep"=w324:i32[], "Applied Current [nA]"=w304:dbl[][][], "Induced Voltage [V]"=w305:dbl[][][], "Voltages OUT"=w307:dbl[], "Compliance exceeded?"=w314:bool)  [unwired: 2 in, 3 out]
                      n164 = property on="Bias On/Off:" class="Bool (strict)"("Blinking"=w314) -> ()  [unwired: 2 in, 2 out]
                      n165 = local write "Ris SMU Current [nA]"(w304) -> ()
                      n166 = Array Size(array=w307) -> (size(s)=w322:i32)
                      n167 = Array Size(array=w324) -> (size(s)=w323:i32)
                      n168 = local write "Ris induced Voltage [V]"(w305) -> ()
                      n169 = for {
                        N: w322 -> [_]
                        tunnel: "No. of readouts" -> [w342]
                        tunnel: w323 -> [w341]
                        tunnel: w304 -> [w340] mode=indexing
                        tunnel: w305 -> [w339] mode=indexing
                        tunnel: w324 -> [w335]
                        tunnel: [w330] -> w313 mode=indexing
                        tunnel: [w329] -> w310 mode=indexing
                        tunnel: [w331] -> w303 mode=indexing
                        tunnel: [w331] -> w299
                        tunnel: [w326] -> w312 mode=indexing
                        tunnel: [w325] -> w309 mode=indexing
                        w338 = T11 0 items=["Least Square", "Least Absolute Residual", "Bisquare"] ("method")
                        w337 = T11 0 items=["Least Square", "Least Absolute Residual", "Bisquare"] ("method")
                        n170 = for {
                          N: w341 -> [_]
                          tunnel: w342 -> [_]
                          tunnel: w340 -> [w348] mode=indexing
                          tunnel: w339 -> [w347] mode=indexing
                          tunnel: [w346] -> w336 mode=indexing
                          tunnel: [w345] -> w334 mode=indexing
                          tunnel: [w344] -> w327 mode=indexing
                          tunnel: [w343] -> w328 mode=indexing
                          n171 = call <vilib>:"Std Deviation and Variance.vi"("X"=w348) -> ("mean"=w346:dbl, "standard deviation"=w344:dbl)  [unwired: 1 in, 1 out]
                          n172 = call <vilib>:"Std Deviation and Variance.vi"("X"=w347) -> ("mean"=w345:dbl, "standard deviation"=w343:dbl)  [unwired: 1 in, 1 out]
                        }
                        n173 = call <vilib>:"Linear Fit.vi"("Y"=w336, "X"=w335, "method"=w338) -> ("slope"=w332:dbl)  [unwired: 8 in, 4 out]
                        n174 = call <vilib>:"Linear Fit.vi"("Y"=w334, "X"=w335, "method"=w337) -> ("slope"=w333:dbl)  [unwired: 8 in, 4 out]
                        n175 = Bundle("Sweep"=w335, w336) -> (w330:cluster{"Sweep":i32[], dbl[]})  [unwired: 1 in]
                        n176 = Bundle("Sweep"=w335, w334) -> (w329:cluster{"Sweep":i32[], dbl[]})  [unwired: 1 in]
                        n177 = formula code="y=1e9/(x1*x2);"("x1"=w332, "x2"=w333) -> ("y"=w331:dbl)
                        n178 = call "XYerrorbars.vi"("XY plot"=w330, "Yerror"=w327) -> ("Y error bars"=w326:cluster{dbl[], dbl[]})  [unwired: 6 in, 2 out]
                        n179 = call "XYerrorbars.vi"("XY plot"=w329, "Yerror"=w328) -> ("Y error bars"=w325:cluster{dbl[], dbl[]})  [unwired: 6 in, 2 out]
                      }
                      n180 = Absolute Value(x=w307) -> (abs(x)=w306:dbl[])
                      n181 = Build Array (concatenate)(w313, w312) -> (w311:cluster{"Sweep":dbl[], dbl[]}[])
                      n182 = Build Array (concatenate)(w310, w309) -> (w308:cluster{"Sweep":dbl[], dbl[]}[])
                      n183 = Bundle(w306, w303) -> (w302:cluster{dbl[], dbl[]})  [unwired: 1 in]
                      n184 = Increment(x=w298) -> (x+1=w297:u32)
                      n185 = call "RisData.vi"("Action"=T2."Write Element", "Array No."=2, "Array Size / Index"=w298, "Data IN"=w299) -> ()  [unwired: 1 in, 2 out]
                      n186 = local write "Imgraph"(w311) -> ()
                      n187 = local write "Vigraph"(w308) -> ()
                      n188 = local write "Risgraph"(w302) -> ()
                      n189 = local write "Current reading No."(w297) -> ()
                    }
                  }
                }
                frame True {
                }
              }
            }
          }
          n190 = Build Array("abort", w244) -> (w248:bool[])
        }
        frame True {
          w350 = FALSE
          # "compliance was exceeded when first voltage applied."
          # "Flag compliance as reason for end of run"
          n191 = local write "STATUS 1"("Run aborted - compliance exceeded.") -> ()
          n192 = Build Array(w350, TRUE, w350, w350) -> (w351:bool[])
        }
      }
      n193 = Search 1D Array(1D array=w236, element=TRUE) -> (index of element=w234:i32)  [unwired: 1 in]
      n194 = Increment(x=w234) -> (x+1=w233:i32)
      n195 = case shown="2" w233 {
        tunnel: ["" "Run ended normally" "Compliance exceeded" "Run aborted - by user" "Run aborted - Ilimit exceeded"] -> w228
        frame ..0 {
        }
        frame 1 {
        }
        frame 2 {
          # "Determine reason for end of run."
        }
        frame 3 {
        }
        frame 4.. {
        }
      }
      n196 = global read "QC_RunInformation.vi" "Run info"() -> (w232:T6)
      n197 = Bundle By Name(cluster=w232, "End of Run comment:"=w228) -> (w227:T6)
      n198 = Concatenate Strings(w228, "\r\n", "RAMPING DOWN VOLTS") -> (w231:string)
      n199 = global write "QC_RunInformation.vi" "Run info"(w227) -> ()
      n200 = local write "STATUS 1"(w231) -> ()
    }
    frame #4 {
      n201 = stacked-sequence {
        frame #0 {
          # "Tie up loose ends. Set volts to zero and switch to standby"
          # "Ramp down volts now"
          n202 = global read "QC_MeasurementSetup.vi" "Ris Measurement Parameters"() -> (w359:T8)
          n203 = Unbundle By Name(w359) -> ("SMU"=w355:refnum<class "SupplyControl.lvclass">, "Bias Supply"=w356:refnum<class "SupplyControl.lvclass">, "Ramp down steps [V]"=w358:dbl, "Ramp down Interval [s]"=w357:i32, "Multimeter"=w369:refnum<class "MultimeterControl.lvclass">, "Switching"=w370:refnum<class "Switching.lvclass">, "Matrix used?"=w371:bool)
          n204 = Multiply(x=w357, y=1000) -> (x*y=w361:i32)
          n205 = local read "Current Volts:"() -> (w364:dbl)
          n206 = call-dynamic "Supply_Stby.vi"("SupplyControl in"=w355) -> ("error out"=w354:errorcluster)  [unwired: 9 in, 1 out]
          n207 = call "SupplyRamp.vi"("error in"=w354, "Requested Voltage"=0.0, "Step Size"=w358, "Step Delay"=w361, "Supply IN"=w356, "Starting Voltage"=w364) -> ("error out"=w366:errorcluster, "Supply OUT"=w365:refnum<class "SupplyControl.lvclass">, "Current Voltage"=w362:dbl)  [unwired: 2 in, 1 out]
          n208 = local write "Current Volts:"(w362) -> ()
          n209 = call-dynamic "Supply_Stby.vi"("error in (no error)"=w366, "SupplyControl in"=w365) -> ("error out"=w367:errorcluster)  [unwired: 8 in, 1 out]
          n210 = call-dynamic "Multimeter_Reset.vi"("error in (no error)"=w367, "MultimeterControl in"=w369) -> ("error out"=w368:errorcluster)  [unwired: 8 in, 1 out]
          n211 = case shown="True" w371 {
            tunnel: w370 -> [_ w376]
            tunnel: w368 -> [_ w375]
            frame False {
            }
            frame True {
              n212 = call-dynamic "MatrixSwitch.vi"("error in (no error)"=w375, "Action"=T3."Reset", "Switching in"=w376) -> ("error out"=w372:errorcluster, "Switching out"=w373:refnum<class "Switching.lvclass">)  [unwired: 6 in, 1 out]
              n213 = call-dynamic "Close.vi"("error in (no error)"=w372, "Switching in"=w373) -> ()  [unwired: 8 in, 2 out]
            }
          }
        }
        frame #1 {
          w381 = 0
          n214 = local write "Bias On/Off:"(FALSE ("Visible")) -> ()
          n215 = local write "Current Volts:"(0.0 ("Current Volts:")) -> ()
          n216 = property on="Quit & Save" class="Bool"("DisabledEnum"=w381) -> ()  [unwired: 2 in, 2 out]
          n217 = property on="quit (no save)" class="Bool"("DisabledEnum"=w381) -> ()  [unwired: 2 in, 2 out]
          n218 = property on="abort" class="Bool (strict)"("DisabledEnum"=2) -> ()  [unwired: 2 in, 2 out]
          n219 = local write "STATUS 1"("Run finished. \nSave data?" ("STATUS 1")) -> ()
        }
        frame #2 {
          n220 = Current VI's Path() -> (path=w383:path)
          n221 = call "SaveJPEG.vi"("Test"="Ris", "File Path Control"=w383) -> ()  [unwired: 1 in, 2 out]
        }
      }
    }
    frame #5 {
      # "Loop and await decision on whether to save or junk data"
      n222 = while {
        tunnel: ["Quit & Save"] -> w393
        tunnel: ["quit (no save)"] -> w392
        stop <- w431 continue-if-true
        n223 = Not Or(1:"quit (no save)", 2:"Quit & Save") -> (0:w431:bool)
      }
      n224 = global read "QC_MeasurementSetup.vi" "Ris Measurement Parameters"() -> (w391:T8)
      n225 = Unbundle By Name(w391) -> ("Temperature Readout"=w390:enum16{"Read Arduino", "Enter manually"}, "Arduino"=w386:refnum<class "ArduinoControl.lvclass">)
      n226 = case shown="\"Read Arduino\"" w390 {
        tunnel: w386 -> [_ w429]
        frame "Enter manually", Default {
        }
        frame "Read Arduino" {
          n227 = call "ArduinoClose.vi"("ArduinoControl in"=w429) -> ()  [unwired: 9 in, 2 out]
        }
      }
      n228 = case shown="True" w392 {
        tunnel: [FALSE w434] -> w394
        frame False {
        }
        frame True {
          n229 = Two Button Dialog(message="Are you sure you don't want to save the data?", 1:"Quit" ("F button name (\"Cancel\")"), 2:"Save data" ("T button name (\"OK\")")) -> (T button?=w434:bool)
        }
      }
      n230 = Or(x=w393, y=w394) -> (x .or. y?=w384:bool)
      n231 = case shown="True" w384 {
        tunnel: w384 -> [_ w428]
        frame False {
        }
        frame True {
          w408 = T2."Read Array" ("Action")
          n232 = local write "STATUS 1"("Saving Data ...") -> ()
          n233 = global read "QC_MeasurementSetup.vi" "Ris Measurement Parameters"() -> (w425:T8)
          n234 = call "RisData.vi"("Action"=w408, "Array No."=u32 1 ("Action")) -> ("Array OUT"=w419:dbl[])  [unwired: 3 in, 1 out]
          n235 = call "RisData.vi"("Action"=w408, "Array No."=u32 2 ("Action")) -> ("Array OUT"=w406:dbl[])  [unwired: 3 in, 1 out]
          n236 = call "RisData.vi"("Action"=w408, "Array No."=u32 0 ("Action")) -> ("Array OUT"=w400:dbl[])  [unwired: 3 in, 1 out]
          n237 = Build Array(w400, w419, w406) -> (w418:dbl[][])
          n238 = call "RisData.vi"("Action"=w408, "Array No."=u32 4 ("Action")) -> ("Array OUT"=w424:dbl[])  [unwired: 3 in, 1 out]
          n239 = call "RisData.vi"("Action"=w408, "Array No."=u32 3 ("Action")) -> ("Array OUT"=w401:dbl[])  [unwired: 3 in, 1 out]
          n240 = Unbundle By Name(w425) -> ("R_is Limit [MOhm]"=w410:dbl, "Number Of Steps"=w397:u32)
          n241 = call <vilib>:"Std Deviation and Variance.vi"("X"=w424) -> ("mean"=w415:dbl)  [unwired: 1 in, 2 out]
          n242 = call <vilib>:"Std Deviation and Variance.vi"("X"=w401) -> ("mean"=w416:dbl)  [unwired: 1 in, 2 out]
          n243 = Transpose 2D Array(2D array=w418) -> (transposed array=w417:dbl[][])
          n244 = local read "Ris induced Voltage [V]"() -> (w404:dbl[][][])
          n245 = local read "Ris SMU Current [nA]"() -> (w405:dbl[][][])
          n246 = call "ScanFeedback.vi"("measurement type"=T5."Ris") -> ("V breakdown"=w412:dbl)  [unwired: 4 in, 4 out]
          n247 = call "SaveDataFile.vi"("Data Array"=w417, "Temperature"=w416, "Humidity"=w415, "Array Titles"="Voltage[V] Current[nA] R_is[MOhm]", "Strip Segment"="") -> ("Path + Filename OUT"=w402:string, "Error Out"=w399:errorcluster)  [unwired: 7 in, 2 out]
          n248 = Absolute Value(x=w412) -> (abs(x)=w411:dbl)
          n249 = Absolute Value(x=w410) -> (abs(x)=w409:dbl)
          n250 = call "SaveRisRawData.vi"("Filename"=w402, "Induced Voltage [V]"=w404, "Volts"=w400, "error in (no error)"=w399, "SMU Current [nA]"=w405, "Data formats"="%010.2f", "Number of data points"=w397) -> ("error out"=w398:errorcluster)  [unwired: 3 in]
          n251 = Greater Or Equal?(x=w411, y=w409) -> (x >= y?=w413:bool)
          n252 = call "WriteLogFile.vi"("Automatic warning"="", "Data File"=w402, "Error In"=w398, "DUT passed?"=w413, "Value TechSpec criteria"=w412, "Files saved?"=w428) -> ()  [unwired: 5 in, 1 out]
        }
      }
      n253 = Select(t="Run finished.\nData saved." ("STATUS 1"), s=w384, f="Run finished.\nData not saved." ("STATUS 1")) -> (s? t:f=w389:string)
      n254 = local write "STATUS 1"(w389) -> ()
      "Done!" <- TRUE
    }
  }
